vi "Post-Build Action Scripting.vi"(5 "Files Generated by Build":path[](array[path]), 6 "Top Level/Always Included VIs":path[](array[path]), 7 "Destination Path":path, 8 "error in (no error)":errorcluster, 9 "Target Name":string, 10 "Build Specification Name":string, 11 "Project Path":path) -> (0 "error out":errorcluster)   [LabVIEW 2020]
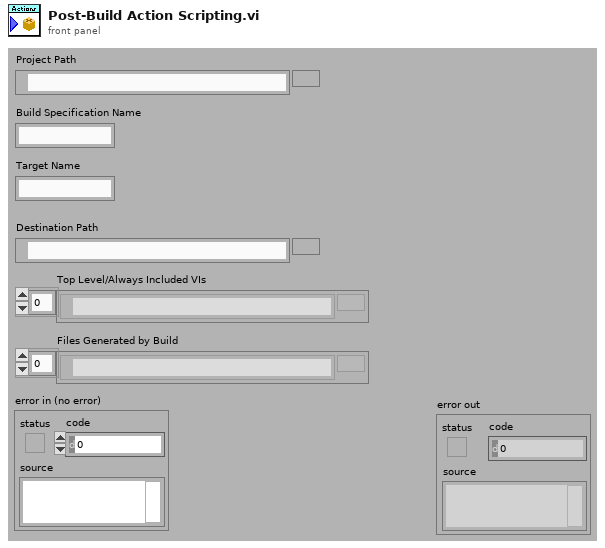
[diagram p1: front panel]
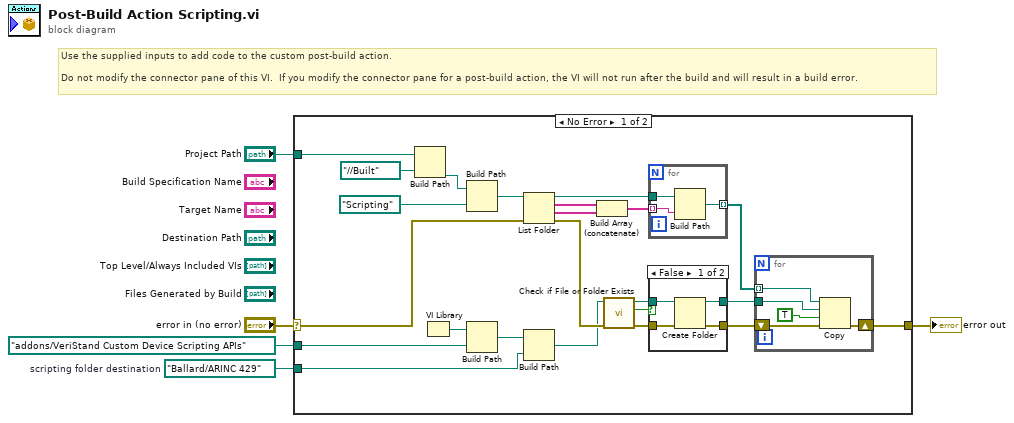
[diagram p0: block diagram]
diagram:
  w3 = path "Ballard/ARINC 429"  # scripting folder destination
  # "Use the supplied inputs to add code to the custom post-build action.\n\nDo not modify the connector pane of this VI.  If you modify the connector pane for a post-build action, the VI will not run after the build and will result in a build error."
  n1 = case shown="No Error" "error in (no error)" {
    selector: "error in (no error)" -> [w6 w43]
    tunnel: [w12 w43] -> w5
    tunnel: "Project Path" -> [w20 _]
    tunnel: w3 -> [w15 _]
    tunnel: path "addons/VeriStand Custom Device Scripting APIs" ("name or relative path") -> [w7 _]
    frame No Error {
      n2 = Build Path(base path=w20, name or relative path=path "../../Built") -> (appended path=w22:path)
      n3 = VI Library() -> (path=w16:path)
      n4 = Build Path(base path=w22, name or relative path=path "Scripting") -> (appended path=w24:path)
      n5 = Build Path(base path=w16, name or relative path=w7) -> (appended path=w14:path)
      n6 = List Folder(path=w24, error in=w6) -> (path out=w25:path, filenames=w10:string[], folder names=w11:string[], error out=w23:errorcluster)  [unwired: 2 in]
      n7 = Build Path(base path=w14, name or relative path=w15) -> (appended path=w13:path)
      n8 = Build Array (concatenate)(w10, w11) -> (w9:string[])
      n9 = call <vilib>:"Check if File or Folder Exists.vi"("error in (no error)"=w23, "path"=w13) -> ("error out"=w26:errorcluster, "file or folder exists?"=w28:bool, "dup path"=w27:path)  [unwired: 7 in]
      n10 = for {
        tunnel: w9 -> [w41] mode=indexing
        tunnel: w25 -> [w42]
        tunnel: [w40] -> w8 mode=indexing
        n11 = Build Path(base path=w42, name or relative path=w41) -> (appended path=w40:path)
      }
      n12 = case shown="False" w28 {
        tunnel: w27 -> [w32 w34]
        tunnel: w26 -> [w31 w33]
        tunnel: [w30 w34] -> w18
        tunnel: [w29 w33] -> w19
        frame False {
          n13 = Create Folder(path (use dialog)=w32, error in=w31) -> (created path=w30:path, error out=w29:errorcluster)  [unwired: 1 in, 1 out]
        }
        frame True {
        }
      }
      n14 = for {
        tunnel: w8 -> [w36] mode=indexing
        shift-right: [w37] -> w12
        shift-left: w19 -> [w38]
        tunnel: w18 -> [w35]
        n15 = Copy(8:w38, 9:TRUE ("overwrite (F)"), 10:w35, 11:w36) -> (0:w37:errorcluster)  [unwired: 1 in, 2 out]
      }
    }
    frame Error {
    }
  }
  "error out" <- w5
